vi "GetOwningStructure.vi"(6 "error in":errorcluster, 9 "Tunnel in":refnum<class "Tunnel.lvclass">) -> (0 "error out":errorcluster, 3 "Tunnel out":refnum<class "Tunnel.lvclass">, 4 "UID":i32)   [LabVIEW 2014, in "Tunnel.lvclass"]
uses:
  Tunnel.lvclass
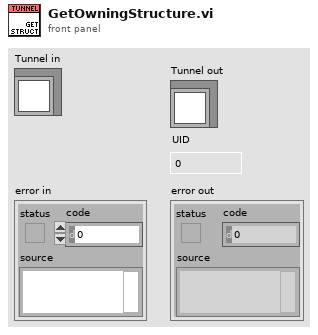
[diagram p1: front panel]
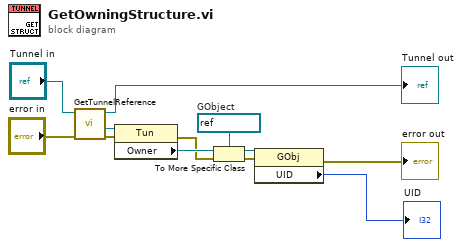
[diagram p0: block diagram]
diagram:
  w6 = refnum<vi> refnum  # GObject
  n1 = call "GetTunnelReference.vi"("error in"="error in", "Tunnel in"="Tunnel in") -> ("error out"=w10:errorcluster, "reference out"=w11:refnum<vi>, "Tunnel out"=→"Tunnel out":refnum<class "Tunnel.lvclass">)  [unwired: 7 in]
  n2 = property class="Tun"(reference=w11, error in=w10) -> (error out=w7:errorcluster, "Owner"=w8:refnum<vi>)  [unwired: 1 out]
  n3 = To More Specific Class(target class=w6, reference=w8, error in=w7) -> (specific class reference=w5:refnum<vi>, error out=w4:errorcluster)
  n4 = property class="GObj"(reference=w5, error in=w4) -> (error out=→"error out":errorcluster, "UID"=→"UID":i32)  [unwired: 1 out]
